vi "主画面.vi"() -> ()   [LabVIEW 2016]
uses:
  API/update/tcp_client_data.ctl
  <vilib>/Utility/miscctls.llb/LVPointTypeDef.ctl
  <vilib>/ActorFramework/Message Enqueuer/Message Enqueuer.lvclass/Message Enqueuer.ctl
  <vilib>/Utility/miscctls.llb/LVRectTypeDef.ctl
  <vilib>/ActorFramework/Message Enqueuer/Enqueue.vi
  <vilib>/ActorFramework/Stop Msg/Stop Msg.lvclass
  C:/Program Files (x86)/National Instruments/LabVIEW 2016/vi.lib/ActorFramework/Message/Message.lvclass
  <vilib>/ActorFramework/Message Priority Queue/Priority Enqueue.vi
  Modbus Slave/main/modbus slave new.vi
  data/FreeMem.dll
  API/update/update.lvlib
  Modbus Slave/MB SLAVE.lvlib
  PLC/PLC.lvlib
  API/OpSignIn/opSignIn.lvlib
  <vilib>/ptbypt/NI_PtbyPt.lvlib
panel:
  out "运行时间":string="运行时间"
  in  "软件升级":bool
  out "data":T1
  out "状态显示":string
  out "ver":string
  in  "打卡请点我！":bool
  out "权限等级 2":enum16{"一级权限", "二级权限", "三级权限", "超级权限"}(ring)
  out "权限等级":string
  out "布尔":bool
  in  "关于":bool
  out "SN":string="SN "
  in  "全屏":T2
  out "站点名称":string="站点名称"
  out "时间显示":string="2017-05-09 10:50:42"
  in  "主画面菜单":T3
  # "水质在线自动监测系统"
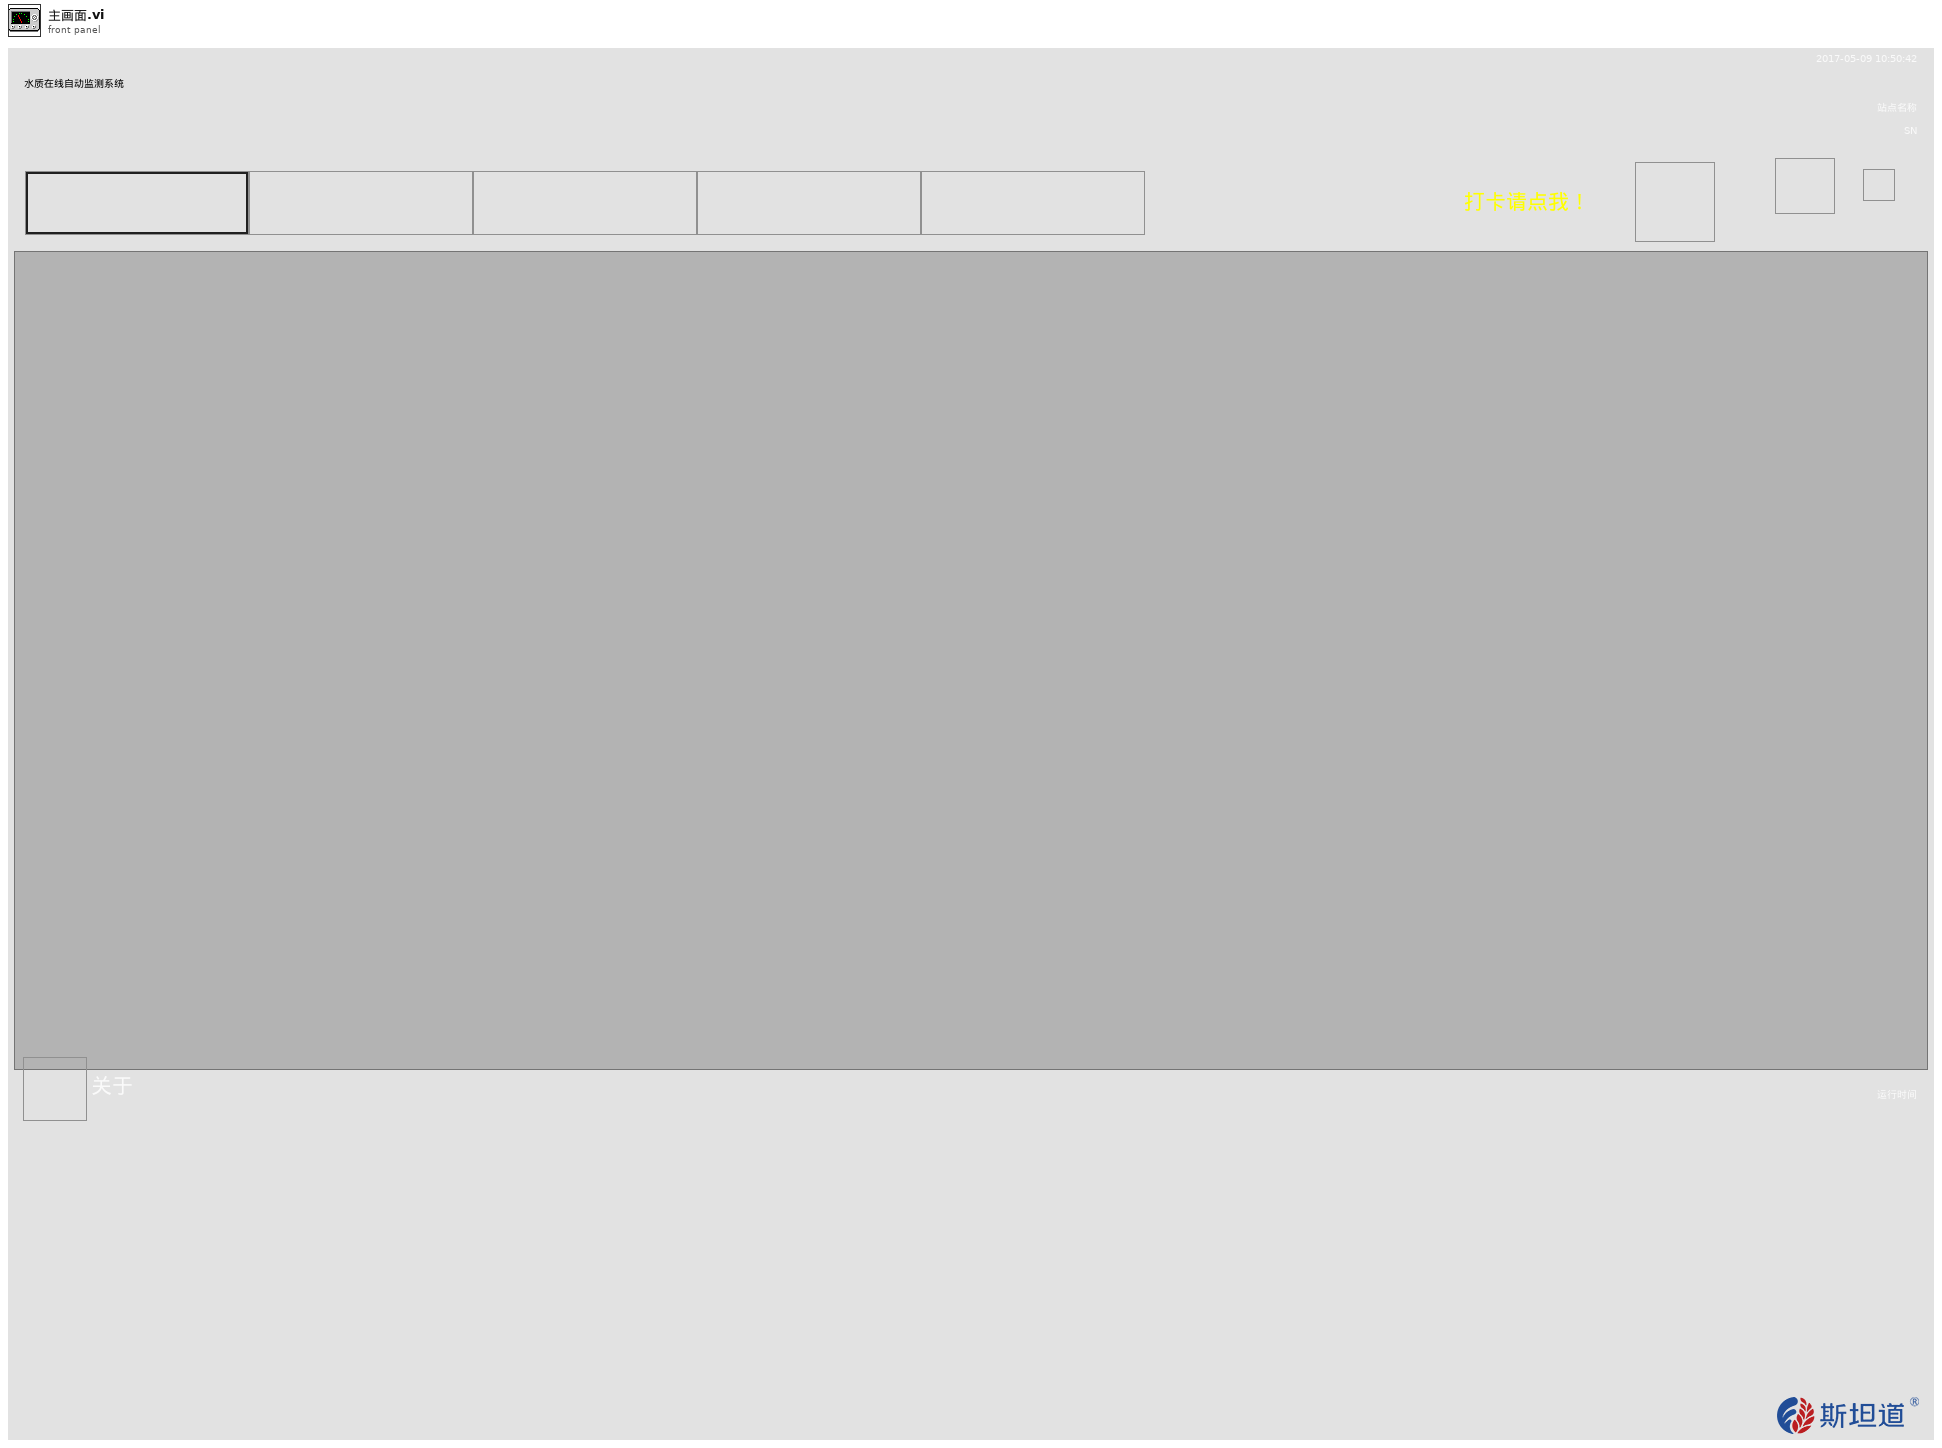
[diagram p1: front panel]
types:
  T1 = typedef "update.lvlib/tcp_client_data.ctl" = cluster{"SPname":string, "MNnumber":string, "Version":string, "state":string, "progress":dbl, "password":string, "data_transmission_Version":string}
  T2 = typedef "全屏按钮.ctl" = bool
  T3 = typedef "主画面单选控件.ctl" = enum32{"首页", "数据查询", "运维调试", "环境动力", "系统设置"}
  T4 = typedef "LVPointTypeDef.ctl" = cluster{"Horizontal":i16, "Vertical":i16}
  T5 = cluster{"时间标识":timestamp, "设备":string, "日志信息":string, "流程参数":string}
  T6 = typedef "设备类型.ctl" = enum16{"微站", "固定站", "浮船"}
  T7 = typedef "系统交互.ctl" = cluster{"运行模式":enum16{"维护模式", "常规模式", "应急模式", "质控模式", "性能测试"}, "运行间隔":i16, "流程运行中":bool, "自动运行启动参数":T8, "SYSTEM Interface.总磷总氮类型":enum16{"单模块", "总磷总氮二合一模块", "氨氮总磷二合一模块"}, "多参数运行间隔":i16, "配水时间":dbl, "沉淀时间":dbl, "清洗时间":dbl, "关键参数改变":bool, "温度告警":bool, "湿度告警":bool, "烟感告警":bool, "水浸告警":bool, "开门告警":bool, "超标留样瓶满告警":bool, "SystemTask":enum16{"停机", "待机", "调试", "水样采集", "沉沙", "进样", "仪表测试分析", "反吹", "清洗", "除藻"}, "PumpState":enum16{"--", "只用泵1", "只用泵2", "双泵交替"}, "除藻选择":enum16{"不开除藻", "开除藻"}, "报警信息":enum16{"无报警", "断电报警", "采样管理欠压（源水泵故障）", "进样管路欠压（进样泵/增加泵故障）"}, "软件升级":bool, "固件升级":enum16{"无", "CODMn", "氨氮", "总磷", "总氮", "CODCr"}, "数据传输软件升级":bool, "数采仪软件版本":string}
  T8 = typedef "启动参数.ctl" = cluster{"氨氮":bool, "总磷":bool, "总氮":bool, "多参数":bool, "CODmn":bool, "CODCr":bool, "氟化物":bool, "超标留样":bool, "重金属":bool, "挥发酚":bool, "综合生物毒性":bool}
  T9 = enum32{"Bad", "Idle", "Run top level", "Running"}
  T10 = typedef "LVRectTypeDef.ctl" = cluster{"Left":i16, "Top":i16, "Right":i16, "Bottom":i16}
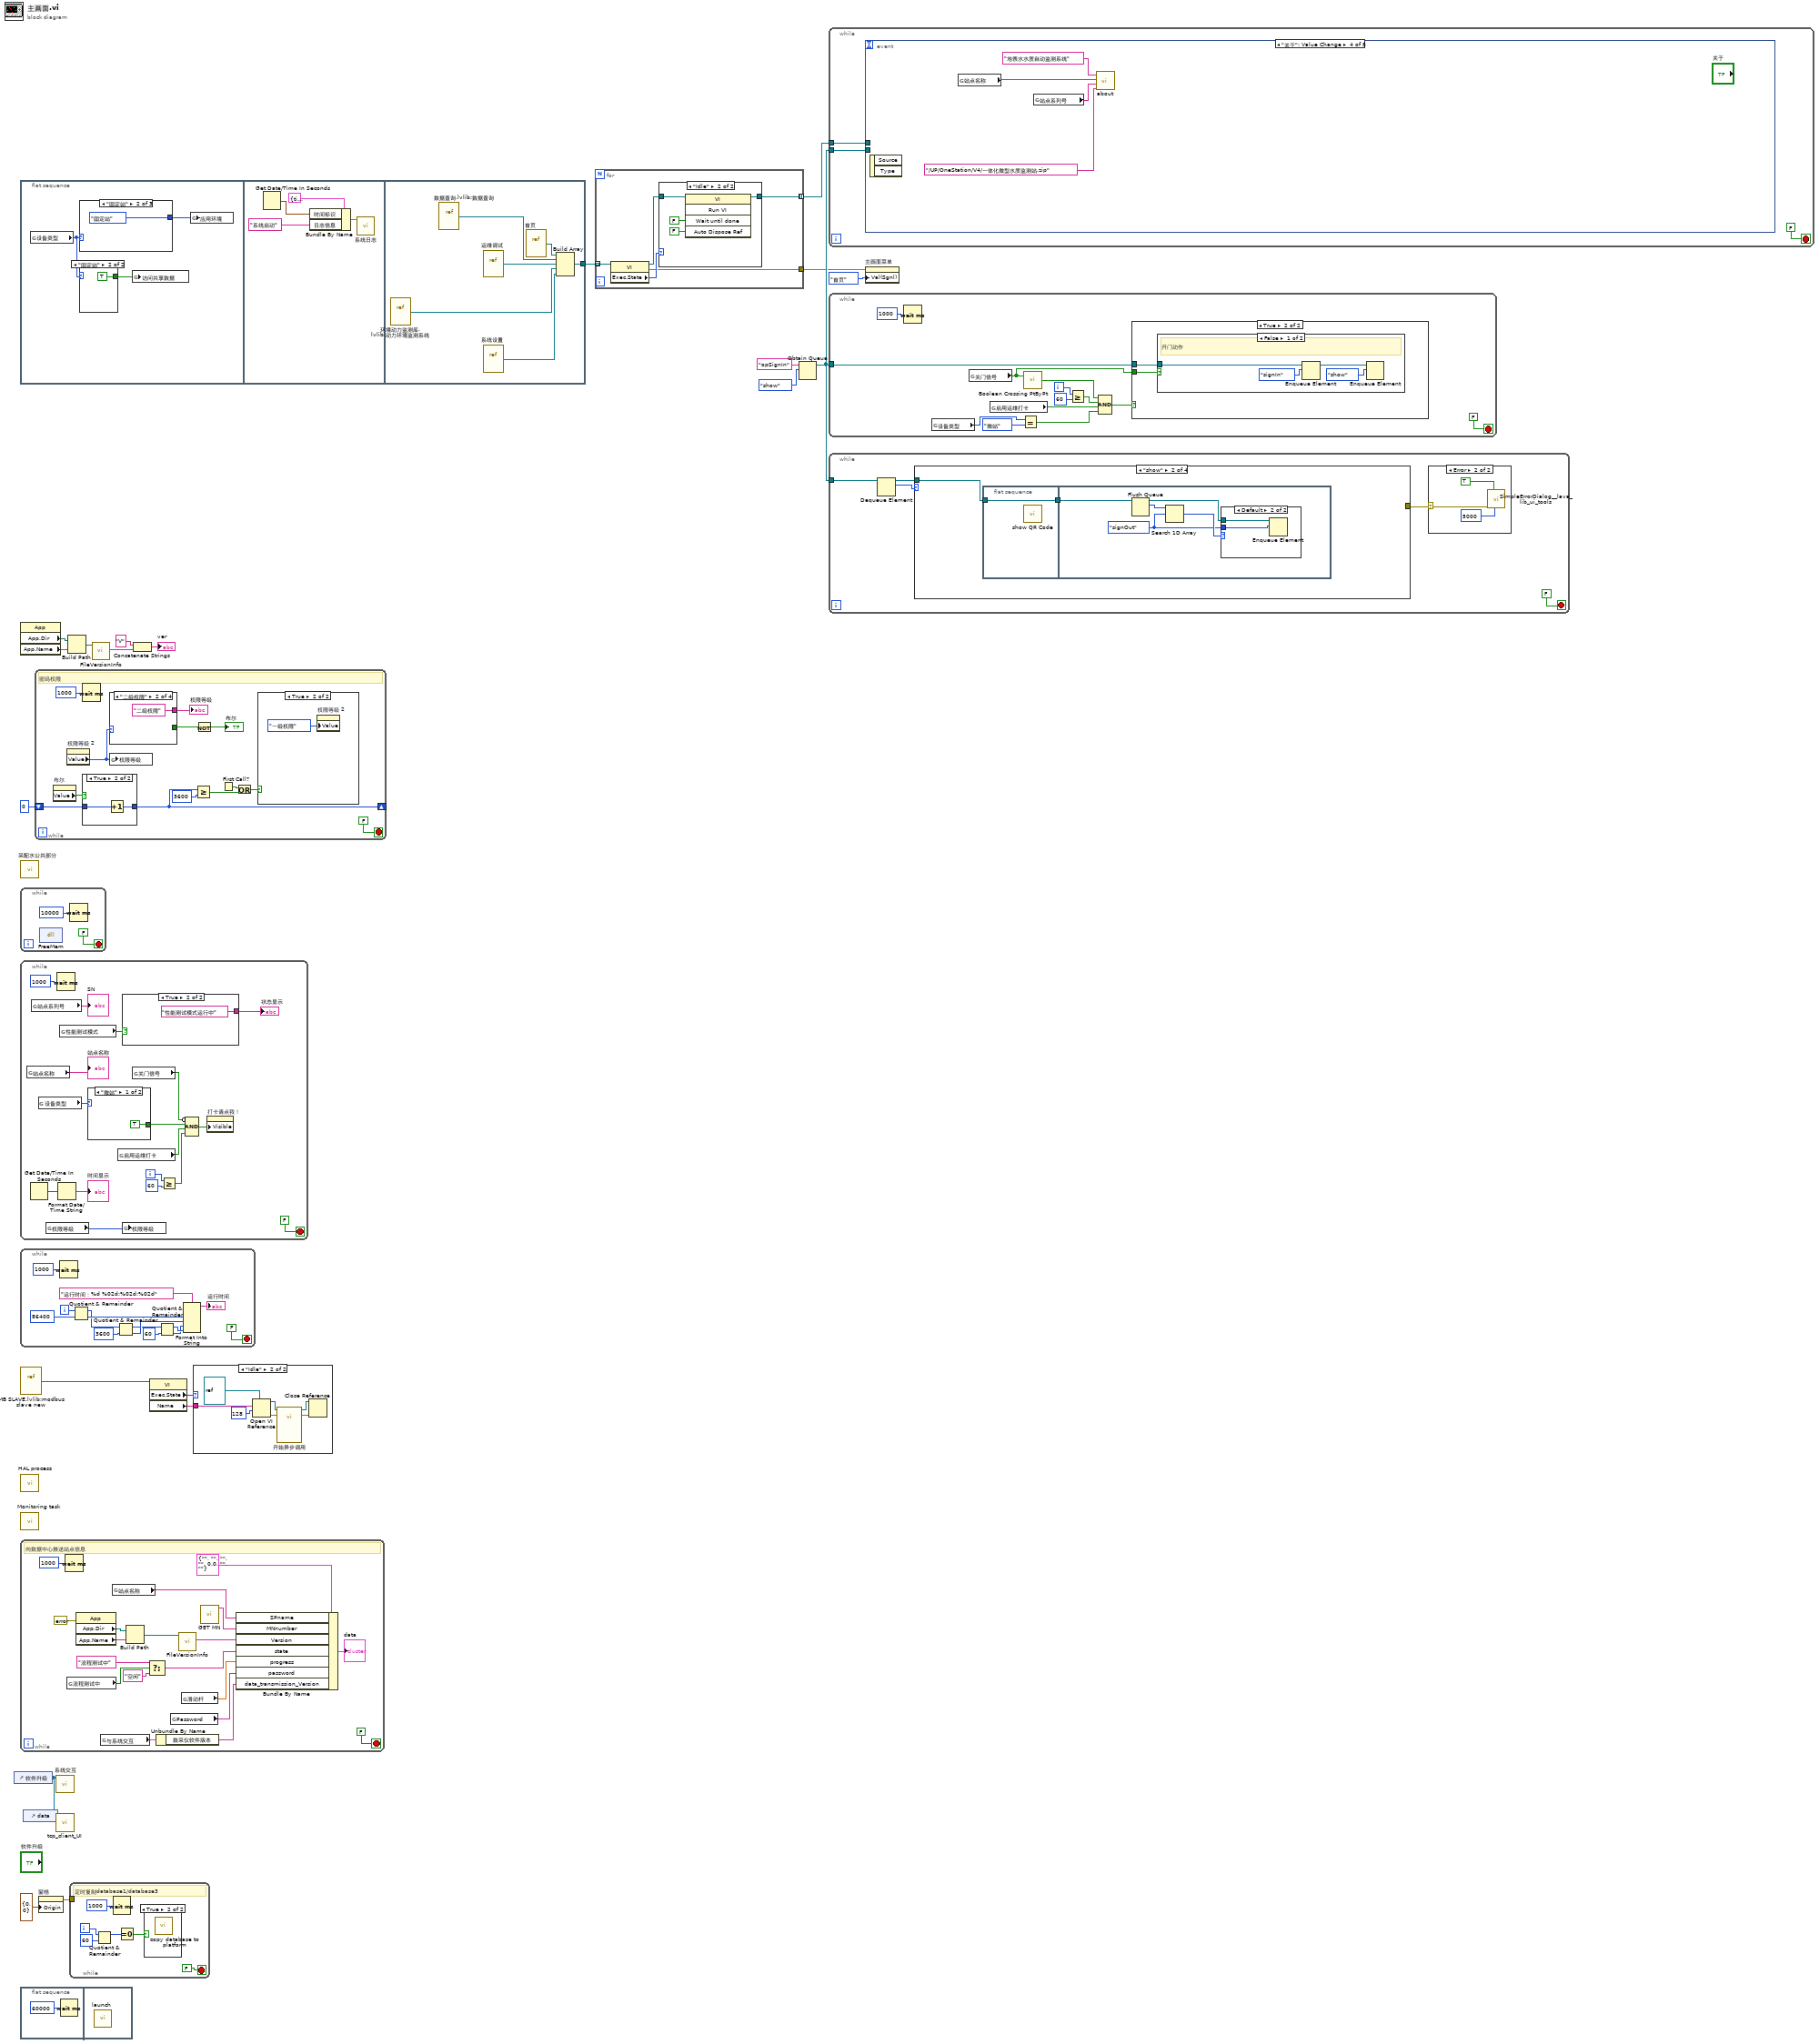
[diagram p0: block diagram]
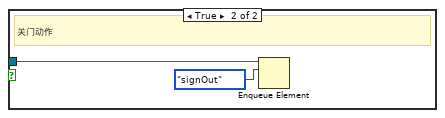
[diagram p3: hidden frame]
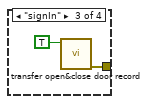
[diagram p7: hidden frame]
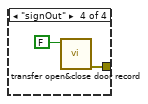
[diagram p8: hidden frame]
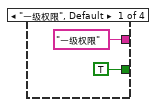
[diagram p9: hidden frame]
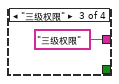
[diagram p10: hidden frame]
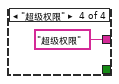
[diagram p11: hidden frame]
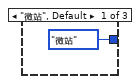
[diagram p17: hidden frame]
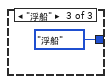
[diagram p18: hidden frame]
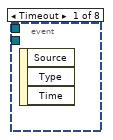
[diagram p20: hidden frame]
diagram:
  n1 = control-ref of="软件升级"() -> (w1:refnum<vi>)
  n2 = flat-sequence {
    tunnel: [w33] -> w15
    frame #0 {
      n3 = global read "系统设置全局变量.vi" "设备类型"() -> (w23:T6)
      n4 = case shown="\"固定站\"" w23 {
        tunnel: [enum16{"固定站", "微站", "浮标", "浮船"}."微站" ("应用环境") enum16{"固定站", "微站", "浮标", "浮船"}."固定站" ("应用环境") enum16{"固定站", "微站", "浮标", "浮船"}."浮船" ("应用环境")] -> w22
        frame "微站", Default {
        }
        frame "固定站" {
        }
        frame "浮船" {
        }
      }
      n5 = case shown="\"固定站\"" w23 {
        tunnel: [_ TRUE ("访问共享数据")] -> w24
        frame "微站", Default {
        }
        frame "固定站" {
        }
      }
      n6 = global write "全局变量.vi" "访问共享数据"(w24) -> ()
      n7 = global write "外部交互全局变量.vi" "应用环境"(w22) -> ()
    }
    frame #1 {
      n8 = Get Date/Time In Seconds() -> (seconds since 1Jan1904=w31:timestamp)
      n9 = Bundle By Name(cluster=T5 {"时间标识"=timestamp(0 s since 1904-01-01), "设备"="系统", "日志信息"="", "流程参数"=""} ("data in"), "时间标识"=w31, "日志信息"="系统启动") -> (w29:T5)
      n10 = call "系统日志.vi"("data in"=w29) -> ()  [unwired: 11 in]
    }
    frame #2 {
      n11 = vi-ref "环境动力监测库.lvlib:动力环境监测系统.vi"() -> (w38:refnum<vi>)
      n12 = vi-ref "数据查询.lvlib:数据查询.vi"() -> (w35:refnum<vi>)
      n13 = vi-ref "运维调试.vi"() -> (w36:refnum<vi>)
      n14 = vi-ref "系统设置.vi"() -> (w37:refnum<vi>)
      n15 = vi-ref "首页.vi"() -> (w34:refnum<vi>)
      n16 = Build Array(w34, w35, w36, w38, w37) -> (w33:refnum<vi>[])
    }
  }
  n17 = property class="App"() -> ("App.Dir"=w8:path, "App.Name"=w6:string)  [unwired: 2 in, 2 out]
  n18 = call "采配水公共部分.vi"() -> ()  [unwired: 12 in]
  n19 = while {
    stop <- FALSE stop-if-true
    n20 = dll-call lib="PTH2|abs CUserslisha\tDocuments\nGitSourcecodeone-station-project-template一体站项目 - V4质控dataFreeMem.dll" fn="FreeMem"() -> ()  [unwired: 4 in, 2 out]
    n21 = Wait (ms)(milliseconds to wait=u32 10000 ("等待时间（毫秒）")) -> ()  [unwired: 1 out]
  }
  n22 = while {
    i -> [w46]
    stop <- FALSE stop-if-true
    n23 = global read "系统设置全局变量.vi" "站点名称"() -> (→"站点名称":string)
    n24 = Get Date/Time In Seconds() -> (seconds since 1Jan1904=w54:timestamp)
    n25 = global read "系统设置全局变量.vi" "站点系列号"() -> (→"SN":string)
    n26 = global read "系统设置全局变量.vi" "设备类型"() -> (w51:T6)
    n27 = global read "非断电保持全局变量.vi" "权限等级"() -> (w52:enum16{"一级权限", "二级权限", "三级权限", "超级权限"})
    n28 = Wait (ms)(milliseconds to wait=u32 1000 ("等待时间（毫秒）")) -> ()  [unwired: 1 out]
    n29 = Format Date/Time String(seconds (now)=w54) -> (date/time string=→"时间显示":string)  [unwired: 2 in]
    n30 = global read "系统设置全局变量.vi" "性能测试模式"() -> (w43:bool)
    n31 = case shown="\"微站\"" w51 {
      tunnel: [TRUE _] -> w50
      frame "微站" {
      }
      frame "固定站", Default {
      }
    }
    n32 = global read "系统设置全局变量.vi" "启用运维打卡"() -> (w48:bool)
    n33 = case shown="True" w43 {
      tunnel: [_ "性能测试模式运行中" ("状态显示")] -> w42
      frame False {
      }
      frame True {
      }
    }
    "状态显示" <- w42
    n34 = global write "外部交互全局变量.vi" "权限等级"(w52) -> ()
    n35 = global read "采配水全局变量.vi" "关门信号"() -> (w47:bool)
    n36 = Greater Or Equal?(x=w46, y=60) -> (x >= y?=w44:bool)
    n37 = Compound Arithmetic op=AND ("复合运算")(invert w47, w50, w48, w44) -> (w49:bool)
    n38 = property on="打卡请点我！" class="Bool (strict)"("Visible"=w49) -> ()  [unwired: 2 in, 2 out]
  }
  n39 = while {
    i -> [w61]
    stop <- FALSE stop-if-true
    n40 = Wait (ms)(milliseconds to wait=u32 1000 ("等待时间（毫秒）")) -> ()  [unwired: 1 out]
    n41 = Quotient & Remainder(x=w61, y=86400) -> (x-y*floor(x/y)=w63:i32, floor(x/y)=w69:i32)
    n42 = Quotient & Remainder(x=w63, y=3600) -> (x-y*floor(x/y)=w65:i32, floor(x/y)=w70:i32)
    n43 = Quotient & Remainder(x=w65, y=60) -> (x-y*floor(x/y)=w72:i32, floor(x/y)=w71:i32)
    n44 = Format Into String(format string="运行时间：%d %02d:%02d:%02d" ("格式字符串"), w69, w70, w71, w72) -> (resulting string=→"运行时间":string)  [unwired: 2 in, 1 out]
  }
  n45 = vi-ref "MB SLAVE.lvlib:modbus slave new.vi"() -> (w20:refnum<vi>)
  n46 = call "HAL process.vi"() -> ()  [unwired: 12 in]
  n47 = call "Monitoring task.vi"() -> ()  [unwired: 12 in]
  n48 = while {
    stop <- FALSE stop-if-true
    # "向数据中心推送站点信息"
    n49 = Wait (ms)(milliseconds to wait=u32 1000 ("等待时间（毫秒）")) -> ()  [unwired: 1 out]
    n50 = global read "系统设置全局变量.vi" "流程测试中"() -> (w82:bool)
    n51 = property class="App"(error in=errorcluster {"status"=FALSE, "code"=0, "source"=""} ("错误输出")) -> ("App.Dir"=w89:path, "App.Name"=w91:string)  [unwired: 1 in, 2 out]
    n52 = global read "modbus slave全局.vi" "与系统交互"() -> (w77:T7)
    n53 = global read "系统设置全局变量.vi" "站点名称"() -> (w74:string)
    n54 = Build Path(base path=w89, name or relative path=w91) -> (appended path=w90:path)
    n55 = Select(t="流程测试中", s=w82, f="空闲") -> (s? t:f=w79:string)
    n56 = Unbundle By Name(w77) -> ("数采仪软件版本"=w76:string)
    n57 = global read "非断电保持全局变量.vi" "Password"() -> (w75:string)
    n58 = call <vilib>:"FileVersionInfo.vi"("Application Path in"=w90) -> ("File Version Info"=w88:string)  [unwired: 7 in, 3 out]
    n59 = global read "更新全局变量.vi" "滑动杆"() -> (w78:dbl)
    n60 = call "GET MN.vi"() -> ("MN"=w92:string)  [unwired: 9 in, 2 out]
    n61 = Bundle By Name(cluster=T1 {"SPname"="", "MNnumber"="", "Version"="", "state"="", "progress"=0.0, "password"="", "data_transmission_Version"=""} ("data"), "SPname"=w74, "MNnumber"=w92, "Version"=w88, "state"=w79, "progress"=w78, "password"=w75, "data_transmission_Version"=w76) -> (→"data":T1)
  }
  n62 = flat-sequence {
    frame #0 {
      n63 = Wait (ms)(milliseconds to wait=u32 60000 ("等待时间（毫秒）")) -> ()  [unwired: 1 out]
    }
    frame #1 {
      n64 = call "launch.vi"() -> ()  [unwired: 12 in]
    }
  }
  n65 = control-ref of="data"() -> (w2:refnum<vi>)
  n66 = while {
    shift-right: [w103] -> _
    shift-left: u32 0 ("y") -> [w105]
    stop <- FALSE stop-if-true
    # "密码权限"
    n67 = property on="布尔" class="Bool (strict)"() -> ("Value"=w97:bool)  [unwired: 2 in, 2 out]
    n68 = property on="权限等级 2" class="Enum (strict)"() -> ("Value"=w94:enum16{"一级权限", "二级权限", "三级权限", "超级权限"})  [unwired: 2 in, 2 out]
    n69 = Wait (ms)(milliseconds to wait=u32 1000 ("等待时间（毫秒）")) -> ()  [unwired: 1 out]
    n70 = case shown="True" w97 {
      tunnel: w105 -> [_ w114]
      tunnel: [_ w113] -> w103
      frame False {
      }
      frame True {
        n71 = Increment(x=w114) -> (x+1=w113:u32)
      }
    }
    n72 = case shown="\"二级权限\"" w94 {
      tunnel: [TRUE _ _ _] -> w100
      tunnel: ["一级权限" "二级权限" "三级权限" "超级权限"] -> w99
      frame "一级权限", Default {
      }
      frame "二级权限" {
      }
      frame "三级权限" {
      }
      frame "超级权限" {
      }
    }
    "权限等级" <- w99
    n73 = global write "非断电保持全局变量.vi" "权限等级"(w94) -> ()
    n74 = Greater Or Equal?(x=w103, y=u32 3600) -> (x >= y?=w101:bool)
    n75 = Not(x=w100) -> (.not. x?=→"布尔":bool)
    n76 = First Call?() -> (First Call?: T/F=w95:bool)
    n77 = Or(x=w95, y=w101) -> (x .or. y?=w96:bool)
    n78 = case shown="True" w96 {
      frame False {
      }
      frame True {
        n79 = property on="权限等级 2" class="Enum (strict)"("Value"=enum16{"一级权限", "二级权限", "三级权限", "超级权限"}."一级权限" ("权限等级")) -> ()  [unwired: 2 in, 2 out]
      }
    }
  }
  n80 = property on="窗格" class="Pane"("Origin"=T4 {"Horizontal"=0, "Vertical"=0} ("原点")) -> (error out=w17:errorcluster)  [unwired: 2 in, 1 out]
  n81 = call "系统交互.vi"("软件升级"=w1) -> ()  [unwired: 11 in]
  n82 = call "tcp_client_UI.vi"("软件升级"=w1, "data"=w2) -> ()  [unwired: 10 in]
  n83 = Build Path(base path=w8, name or relative path=w6) -> (appended path=w7:path)
  n84 = while {
    tunnel: w17 -> [_]
    i -> [w118]
    stop <- FALSE stop-if-true
    # "定时复制database1/database3"
    n85 = Quotient & Remainder(x=w118, y=60) -> (x-y*floor(x/y)=w116:i32)  [unwired: 1 out]
    n86 = Wait (ms)(milliseconds to wait=u32 1000 ("等待时间（毫秒）")) -> ()  [unwired: 1 out]
    n87 = Equal To 0?(x=w116) -> (x = 0?=w115:bool)
    n88 = case shown="True" w115 {
      frame False {
      }
      frame True {
        n89 = call "copy database to platform.vi"() -> ()  [unwired: 12 in]
      }
    }
  }
  n90 = call <vilib>:"FileVersionInfo.vi"("Application Path in"=w7) -> ("File Version Info"=w5:string)  [unwired: 7 in, 3 out]
  n91 = Concatenate Strings("V" ("字符串"), w5) -> (→"ver":string)
  n92 = property class="VI"(reference=w20) -> ("Exec.State"=w19:T9, "Name"=w18:string)  [unwired: 1 in, 2 out]
  n93 = case shown="\"Idle\"" w19 {
    tunnel: w18 -> [_ w121]
    frame "Bad", Default {
    }
    frame "Idle" {
      n94 = Open VI Reference(type specifier VI Refnum (for type only)=refnum<vi> refnum, vi path=w121, options=128 ("选项")) -> (vi reference=w123:refnum<vi>, error out=w126:errorcluster)  [unwired: 3 in]
      n95 = call-by-ref "开始异步调用"(reference=w123, error in=w126) -> (reference out=w125:refnum<vi>, error out=w127:errorcluster)  [unwired: 12 in]
      n96 = Close Reference(reference=w125, error in (no error)=w127) -> ()  [unwired: 1 out]
    }
  }
  n97 = for {
    tunnel: w15 -> [w132] mode=indexing
    tunnel: [w129] -> w9 mode=indexing
    tunnel: [w128] -> w10
    n98 = property class="VI"(reference=w132) -> (reference out=w130:refnum<vi>, error out=w128:errorcluster, "Exec.State"=w131:T9)  [unwired: 1 in]
    n99 = case shown="\"Idle\"" w131 {
      tunnel: w130 -> [w133 w135]
      tunnel: [w133 w134] -> w129
      frame "Bad", Default {
      }
      frame "Idle" {
        n100 = invoke class="VI" method="Run VI"(reference=w135, "Wait until done"=FALSE ("结束前等待"), "Auto Dispose Ref"=FALSE ("自动销毁引用")) -> (reference out=w134:refnum<vi>)  [unwired: 2 in, 4 out]
      }
    }
  }
  n101 = Obtain Queue(name (unnamed)="opSignIn" ("名称（未命名）"), element data type=enum16{"show", "signIn", "signOut"}."show" ("枚举")) -> (queue out=w12:refnum<queue>)  [unwired: 3 in, 2 out]
  n102 = while {
    tunnel: w12 -> [w139]
    tunnel: w9 -> [w138]
    stop <- FALSE stop-if-true
    n103 = event shown="[3] \"关于\": Value Change" {
      selector: _ -> [_ _ _ _ _ _ _ _]
      dyn-events: _ -> [_ _ _ _ _ _ _ _]
      timeout: _ -> [_ _ _ _ _ _ _ _]
      tunnel: w139 -> [_ _ _ _ _ _ _ w181]
      tunnel: w138 -> [_ _ _ _ w154 _ _ _]
      event Timeout {
        n104 = event-data() -> ()  [unwired: 1 in, 3 out]
      }
      event "布尔": Mouse Down {
        n105 = event-data() -> ("CtlRef"=w142:refnum<vi>)  [unwired: 1 in, 5 out]
        n106 = property class="Bool (strict)"(reference=w142) -> ("Value"=w141:bool)  [unwired: 1 in, 2 out]
        n107 = case shown="False" w141 {
          frame False {
            n108 = global read "系统设置全局变量.vi" "权限密码"() -> (w145:u32[])
            n109 = property on="权限等级 2" class="Enum (strict)"() -> ("Value"=w143:enum16{"一级权限", "二级权限", "三级权限", "超级权限"})  [unwired: 2 in, 2 out]
            n110 = call "密码权限设置.vi"("权限输入"=w143, "权限密码"=w145) -> ("权限输出"=w144:enum16{"一级权限", "二级权限", "三级权限", "超级权限"})  [unwired: 9 in]
            n111 = property on="权限等级 2" class="Enum (strict)"("Value"=w144) -> ()  [unwired: 2 in, 2 out]
          }
          frame True {
            "权限等级 2" <- enum16{"一级权限", "二级权限", "三级权限", "超级权限"}."一级权限" ("权限等级")
          }
        }
      }
      event "权限等级": Mouse Down {
        n112 = event-data() -> ()  [unwired: 1 in, 6 out]
        n113 = global read "系统设置全局变量.vi" "权限密码"() -> (w149:u32[])
        n114 = property on="权限等级 2" class="Enum (strict)"() -> ("Value"=w148:enum16{"一级权限", "二级权限", "三级权限", "超级权限"})  [unwired: 2 in, 2 out]
        n115 = call "密码权限设置.vi"("权限输入"=w148, "权限密码"=w149) -> ("权限输出"=w147:enum16{"一级权限", "二级权限", "三级权限", "超级权限"})  [unwired: 9 in]
        n116 = property on="权限等级 2" class="Enum (strict)"("Value"=w147) -> ()  [unwired: 2 in, 2 out]
      }
      event "关于": Value Change {
        n117 = event-data() -> ()  [unwired: 1 in, 2 out]
        n118 = global read "系统设置全局变量.vi" "站点名称"() -> (w150:string)
        n119 = global read "系统设置全局变量.vi" "站点系列号"() -> (w153:string)
        n120 = call "about.vi"("更新包远端地址"="/UP/OneStation/V4/一体化微型水质监测站.zip", "SN输入"=w153, "站点名称输入"=w150, "应用程序名称输入"="地表水水质自动监测系统") -> ()  [unwired: 8 in]
      }
      event Value Change {
        n121 = event-data() -> ()  [unwired: 1 in, 1 out]
        n122 = invoke on="子面板" class="SubPnl" method="Remove VI"() -> (error out=w155:errorcluster)  [unwired: 3 in, 2 out]
        n123 = Index Array(array=w154, index="主画面菜单") -> (element=w156:refnum<vi>)
        n124 = invoke on="子面板" class="SubPnl" method="Insert VI"(error in=w155, "VI Ref"=w156) -> ()  [unwired: 2 in, 4 out]
      }
      event Panel Close? {
        n125 = event-data() -> ()  [unwired: 1 in, 4 out]
        n126 = Two Button Dialog(message="请再次确认是否关闭！" ("消息")) -> (T button?=w159:bool)  [unwired: 2 in]
        n127 = case shown="True" w159 {
          tunnel: [TRUE ("放弃？") _] -> w158
          frame False {
          }
          frame True {
            n128 = flat-sequence {
              frame #0 {
                n129 = Get Date/Time In Seconds() -> (seconds since 1Jan1904=w164:timestamp)
                n130 = Bundle By Name(cluster=T5 {"时间标识"=timestamp(0 s since 1904-01-01), "设备"="系统", "日志信息"="", "流程参数"=""} ("data in"), "时间标识"=w164, "日志信息"="系统关闭") -> (w162:T5)
                n131 = call "系统日志.vi"("data in"=w162) -> ()  [unwired: 11 in]
              }
              frame #1 {
                n132 = global read "工况数据接口全局.vi" "Actor's Enqueuer"() -> (w166:refnum<class "Message Enqueuer.lvclass">)
                n133 = call <vilib>:"Send Normal Stop.vi"("Message Enqueuer"=w166) -> ()  [unwired: 10 in, 1 out]
              }
              frame #2 {
                n134 = call "stop daemon.vi"() -> ()  [unwired: 11 in, 1 out]
              }
              frame #3 {
                n135 = call "Force Quit LabVIEW.vi"() -> ()  [unwired: 10 in, 2 out]
              }
              frame #4 {
                n136 = Quit LabVIEW(quit? (T)=TRUE ("退出？(T)")) -> ()
              }
            }
          }
        }
        n137 = event-data("Discard?"=w158) -> ()  [unwired: 1 in, 1 out]
      }
      event Value Change {
        n138 = event-data() -> ("NewVal"=w174:T2)  [unwired: 1 in, 5 out]
        n139 = case shown="True" w174 {
          tunnel: [w176 w179] -> w173
          tunnel: [T10 {"Left"=0, "Top"=0, "Right"=1920, "Bottom"=1080} ("前面板窗口:窗口边界") T10 {"Left"=0, "Top"=0, "Right"=1920, "Bottom"=1008} ("前面板窗口:窗口边界")] -> w168
          tunnel: [_ TRUE] -> w172
          frame False {
            w176 = u8 1 items=["AutoHide"=1, "AlwaysOnTop"=2] ("Operation")
          }
          frame True {
            w179 = u8 2 items=["AutoHide"=1, "AlwaysOnTop"=2] ("Operation")
          }
        }
        n140 = property class="VI"("Front Panel.TitleBarVis"=w172, "Front Panel.WinBounds"=w168) -> (error out=w170:errorcluster)  [unwired: 2 in, 1 out]
        n141 = property on="窗格" class="Pane"(error in=w170, "Origin"=T4 {"Horizontal"=0, "Vertical"=0} ("原点")) -> (error out=w169:errorcluster)  [unwired: 1 in, 1 out]
        n142 = call "AutoHide Windows Taskbar.vi"("error in (no error)"=w169, "Operation"=w173) -> ()  [unwired: 5 in, 1 out]
      }
      event "打卡请点我！": Value Change {
        n143 = event-data() -> ()  [unwired: 1 in, 6 out]
        n144 = Enqueue Element(queue=w181, element=enum16{"show", "signIn", "signOut"}."show" ("元素")) -> ()  [unwired: 2 in, 3 out]
      }
    }
  }
  n145 = while {
    tunnel: w12 -> [w189]
    i -> [w194]
    stop <- FALSE stop-if-true
    n146 = Wait (ms)(milliseconds to wait=u32 1000 ("等待时间（毫秒）")) -> ()  [unwired: 1 out]
    n147 = global read "系统设置全局变量.vi" "设备类型"() -> (w184:T6)
    n148 = global read "采配水全局变量.vi" "关门信号"() -> (w188:bool)
    n149 = global read "系统设置全局变量.vi" "启用运维打卡"() -> (w185:bool)
    n150 = Equal?(x=w184, y=设备类型."微站") -> (x = y?=w182:bool)
    n151 = call <vilib>:"Boolean Crossing PtByPt.vi"("input"=w188) -> ("crossing"=w192:bool)  [unwired: 2 in]
    n152 = Greater Or Equal?(x=w194, y=60) -> (x >= y?=w191:bool)
    n153 = Compound Arithmetic op=AND ("复合运算")(w192, w191, w185, w182) -> (w190:bool)
    n154 = case shown="True" w190 {
      tunnel: w189 -> [_ w196]
      tunnel: w188 -> [_ w195]
      frame False {
      }
      frame True {
        n155 = case shown="False" w195 {
          tunnel: w196 -> [w200 w202]
          frame False {
            # "开门动作"
            n156 = Enqueue Element(queue=w200, element=enum16{"show", "signIn", "signOut"}."signIn" ("元素")) -> (queue out=w198:refnum<queue>)  [unwired: 2 in, 2 out]
            n157 = Enqueue Element(queue=w198, element=enum16{"show", "signIn", "signOut"}."show" ("元素")) -> ()  [unwired: 2 in, 3 out]
          }
          frame True {
            # "关门动作"
            n158 = Enqueue Element(queue=w202, element=enum16{"show", "signIn", "signOut"}."signOut" ("元素")) -> ()  [unwired: 2 in, 3 out]
          }
        }
      }
    }
  }
  n159 = while {
    tunnel: w12 -> [w206]
    stop <- FALSE stop-if-true
    n160 = Dequeue Element(queue=w206) -> (queue out=w204:refnum<queue>, element=w205:enum16{"show", "signIn", "signOut"})  [unwired: 2 in, 2 out]
    n161 = case shown="\"show\"" w205 {
      tunnel: [_ _ w221 w223] -> w203
      tunnel: w204 -> [_ w212 _ _]
      frame Default {
      }
      frame "show" {
        n162 = flat-sequence {
          tunnel: w212 -> [w213]
          tunnel: [w213] -> w211
          tunnel: w211 -> [w218]
          frame #0 {
            n163 = call "show QR Code.vi"() -> ()  [unwired: 12 in]
          }
          frame #1 {
            w214 = enum16{"show", "signIn", "signOut"}."signOut" ("元素")
            n164 = Flush Queue(queue=w218) -> (queue out=w216:refnum<queue>, remaining elements=w217:enum16{"show", "signIn", "signOut"}[])  [unwired: 1 in, 1 out]
            n165 = Search 1D Array(1D array=w217, element=w214) -> (index of element=w215:i32)  [unwired: 1 in]
            n166 = case shown="Default" w215 {
              tunnel: w216 -> [_ w220]
              tunnel: w214 -> [_ w219]
              frame -1 {
              }
              frame Default {
                n167 = Enqueue Element(queue=w220, element=w219) -> ()  [unwired: 2 in, 3 out]
              }
            }
          }
        }
      }
      frame "signIn" {
        n168 = call "transfer open&close door record.vi"("isOpenDoor"=TRUE) -> ("error out"=w221:errorcluster)  [unwired: 9 in, 1 out]
      }
      frame "signOut" {
        n169 = call "transfer open&close door record.vi"("isOpenDoor"=FALSE) -> ("error out"=w223:errorcluster)  [unwired: 9 in, 1 out]
      }
    }
    n170 = case shown="Error" w203 {
      selector: w203 -> [_ w208]
      frame No Error {
      }
      frame Error {
        n171 = call <vilib>:"SimpleErrorDialog__lava_lib_ui_tools.vi"("Timeout (-1)"=5000, "Blacken (F)"=TRUE, "dialog error"=w208) -> ()  [unwired: 7 in, 2 out]
      }
    }
  }
  n172 = property on="主画面菜单" class="RadioBtnsControl (strict)"(error in=w10, "Val(Sgnl)"=主画面单选控件."首页" ("值(信号)")) -> ()  [unwired: 1 in, 2 out]
